vi "Forces Set.vi"(8 "error in (no error)":errorcluster, 10 "Force (N)":T1) -> (0 "error out":errorcluster)   [LabVIEW 2021, in "Haptic Prog Interface.lvlib"]
doc: "Returns the forces of the haptic pen in N.\n\n<b>Force:</b> Accepts a cluster of the x, y, and z forces to be applied to the pen (in units of N).\n*Note: The pen must be ran in custom mode (via the start VI) for this to work."
uses:
  Haptic Prog Interface.lvlib
  Haptic-Programming-Interface/src/x64/Debug/Haptic Programming Interface.dll
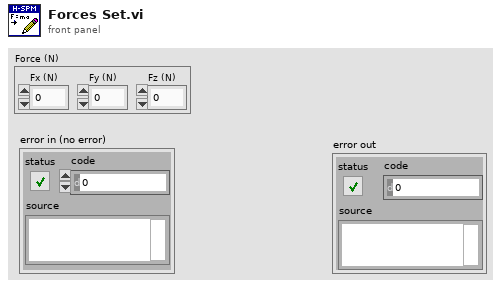
[diagram p1: front panel]
types:
  T1 = cluster{"Fx (N)":dbl, "Fy (N)":dbl, "Fz (N)":dbl}
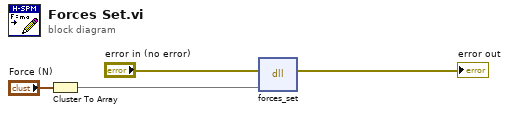
[diagram p0: block diagram]
diagram:
  n1 = Cluster To Array(cluster="Force (N)") -> (array=w1:dbl[])
  n2 = dll-call lib="C:/Users/cjwel/Documents/GitHub/Haptic-Programming-Interface/src/x64/Debug/Haptic Programming Interface.dll" fn="forces_set"(error in="error in (no error)", "input"=w1) -> (error out=→"error out":errorcluster)  [unwired: 4 in, 1 out]
